vi "SyncLoop.vi"(8 "error in (no error)":errorcluster, 11 "NiPxi6682 in":refnum<class "NiPxi6682.lvclass">) -> (0 "error out":errorcluster, 1 "Locked":bool, 2 "Time Ref Offset (ns)":dbl format="%#_12f", 3 "NiPxi6682 out":refnum<class "NiPxi6682.lvclass">, 4 "Lost Lock":bool, 6 "ObtainLock":bool)   [LabVIEW 2014, in "SyncPlugins.lvlib" / "NiPxi6682.lvclass"]
uses:
  NiPxi6682.lvclass
  SyncPluginBase/SyncPluginBase.lvclass/SyncPluginBase.ctl
  NiPxi6682.lvclass/NiPxi6682.ctl
  SyncPluginBase/Accessors/Write Run.vi
  SyncPluginBase/Accessors/Write LostLock.vi
  SyncPluginBase/Accessors/Write Locked.vi
  Accessors/Read NiSyncHandle.vi
  Accessors/Read 1PPS.vi
  Accessors/Read SysRef.vi
  SyncPluginBase/Accessors/Write PPSTime.vi
  SyncPluginBase/Accessors/Read Run.vi
  Accessors/Read clkDiscSession.vi
  SyncPluginBase/Accessors/Read Locked.vi
  <instrlib>/niSync/niSync.llb/niSync Read Trigger Time Stamp (Single).vi
  <resource>/objmgr/niflexriosae.rc
panel:
  out "time stamp out":timestamp format="%^<%.3X\n%x>T"
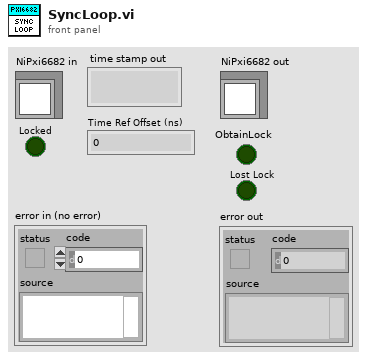
[diagram p1: front panel]
types:
  T1 = typedef "_clkDisc_session.ctl" = variant
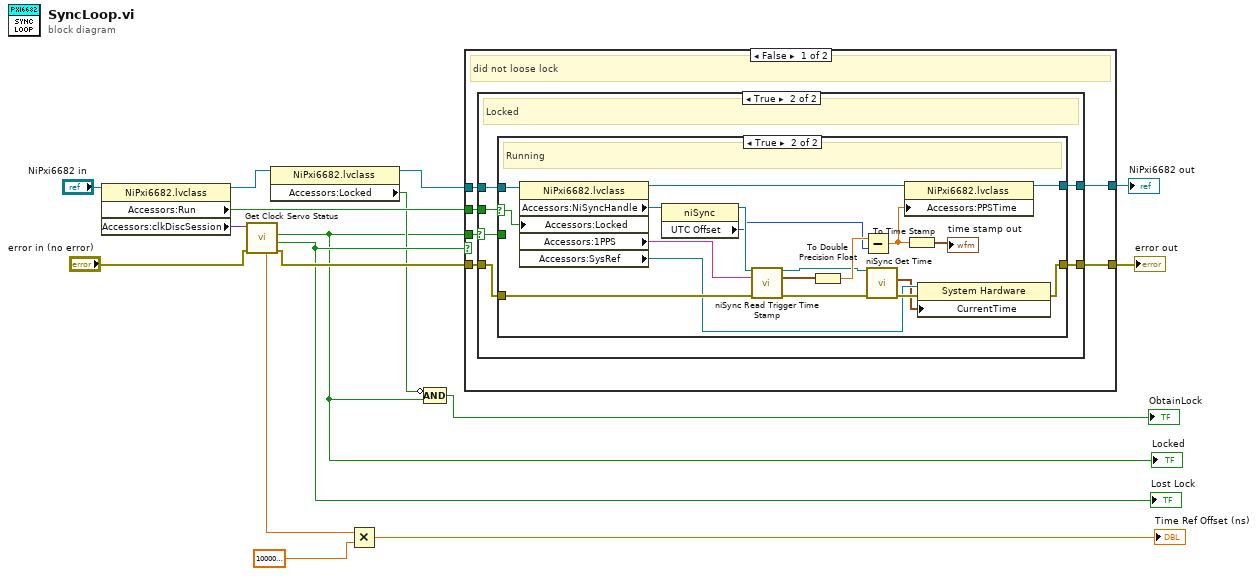
[diagram p0: block diagram]
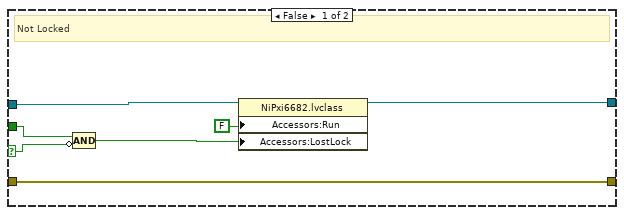
[diagram p2: hidden frame]
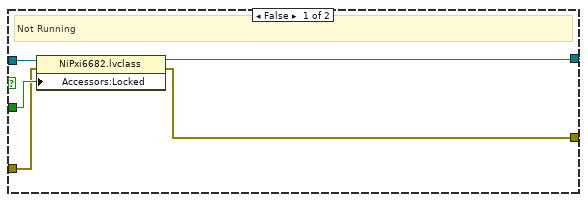
[diagram p3: hidden frame]
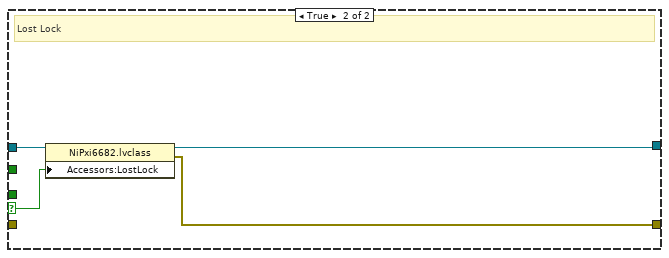
[diagram p4: hidden frame]
diagram:
  n1 = property class="NiPxi6682.lvclass"(reference="NiPxi6682 in") -> (reference out=w5:refnum<class "NiPxi6682.lvclass">, "Accessors:Run"=w14:bool, "Accessors:clkDiscSession"=w15:T1)  [unwired: 1 in, 1 out]
  n2 = call <userlib>:"Get Clock Servo Status.vi"("clkDisc session (in)"=w15, "error out"="error in (no error)") -> ("Calculated Time Reference Offset"=w10:dbl, "Servo Locked"=w2:bool, "Servo Lock Lost"=w6:bool, "error (out)"=w11:errorcluster)  [unwired: 2 in, 1 out]
  "Locked" <- w2
  "Lost Lock" <- w6
  n3 = property class="NiPxi6682.lvclass"(reference=w5) -> (reference out=w4:refnum<class "NiPxi6682.lvclass">, "Accessors:Locked"=w3:bool)  [unwired: 1 in, 1 out]
  n4 = Multiply(x=w10, y=1000000000.0) -> (x*y=→"Time Ref Offset (ns)":dbl)
  n5 = Compound Arithmetic op=AND(invert w3, w2) -> (→"ObtainLock":bool)
  n6 = case shown="False" w6 {
    selector: w6 -> [_ w62]
    tunnel: w4 -> [w22 w63]
    tunnel: w14 -> [w21 _]
    tunnel: [w20 w60] -> w13
    tunnel: w11 -> [w19 _]
    tunnel: w2 -> [w18 _]
    tunnel: [w17 w61] -> w7
    frame False {
      # "did not loose lock"
      n7 = case shown="True" w18 {
        selector: w18 -> [w24 w30]
        tunnel: w22 -> [w29 w34]
        tunnel: [w28 w33] -> w17
        tunnel: w21 -> [w25 w35]
        tunnel: [w26 w32] -> w20
        tunnel: w19 -> [w26 w31]
        frame False {
          # "Not Locked"
          n8 = Compound Arithmetic op=AND(w25, invert w24) -> (w23:bool)
          n9 = property class="NiPxi6682.lvclass"(reference=w29, "Accessors:Run"=FALSE ("Run"), "Accessors:LostLock"=w23) -> (reference out=w28:refnum<class "NiPxi6682.lvclass">)  [unwired: 1 in, 1 out]
        }
        frame True {
          # "Locked"
          n10 = case shown="True" w35 {
            selector: w35 -> [_ w57]
            tunnel: [w39 w53] -> w33
            tunnel: w34 -> [w40 w59]
            tunnel: [w37 w41] -> w32
            tunnel: w31 -> [w36 w56]
            tunnel: w30 -> [w38 _]
            frame False {
              # "Not Running"
              n11 = property class="NiPxi6682.lvclass"(reference=w40, error in=w36, "Accessors:Locked"=w38) -> (reference out=w39:refnum<class "NiPxi6682.lvclass">, error out=w37:errorcluster)
            }
            frame True {
              # "Running"
              n12 = property class="NiPxi6682.lvclass"(reference=w59, "Accessors:Locked"=w57) -> (reference out=w58:refnum<class "NiPxi6682.lvclass">, "Accessors:NiSyncHandle"=w55:refnum<k15>, "Accessors:1PPS"=w54:tag, "Accessors:SysRef"=w43:refnum<k20>)  [unwired: 1 in, 1 out]
              n13 = property class="niSync"(reference=w55) -> (reference out=w52:refnum<k15>, "UTC Offset"=w49:i32)  [unwired: 1 in, 1 out]
              n14 = call-poly <instrlib>:"niSync Read Trigger Time Stamp.vi"("instrument handle"=w52, "terminal"=w54, "error in (no error)"=w56) -> ("instrument handle out"=w45:refnum<k15>, "time stamp out"=w51:timestamp, "error out"=w46:errorcluster)  [unwired: 9 in, 1 out]
              n15 = To Double Precision Float(number=w51) -> (double precision float=w50:dbl)
              n16 = Subtract(x=w50, y=w49) -> (x-y=w47:dbl)
              n17 = call <instrlib>:"niSync Get Time.vi"("error in (no error)"=w46, "instrument handle"=w45) -> ("error out"=w44:errorcluster, "time"=w42:timestamp)  [unwired: 5 in, 1 out]
              n18 = property class="NiPxi6682.lvclass"(reference=w58, "Accessors:PPSTime"=w47) -> (reference out=w53:refnum<class "NiPxi6682.lvclass">)  [unwired: 1 in, 1 out]
              n19 = To Time Stamp(1:w47) -> (0:→"time stamp out":timestamp)
              n20 = property class="System Hardware"(reference=w43, error in=w44, "CurrentTime"=w42) -> (error out=w41:errorcluster)  [unwired: 1 out]
            }
          }
        }
      }
    }
    frame True {
      # "Lost Lock"
      n21 = property class="NiPxi6682.lvclass"(reference=w63, "Accessors:LostLock"=w62) -> (reference out=w61:refnum<class "NiPxi6682.lvclass">, error out=w60:errorcluster)  [unwired: 1 in]
    }
  }
  "error out" <- w13
  "NiPxi6682 out" <- w7
